vi "choosePathDS.vi"(8 "error in (no error)":errorcluster, 10 "ImagesTaken":i32, 11 "Pixelfly in":refnum<class "PixelflySA.lvclass">) -> (0 "error out":errorcluster, 2 "paths":path[](array[path]), 3 "Pixelfly out":refnum<class "PixelflySA.lvclass">)   [LabVIEW 2009, in "PixelflySA.lvclass"]
uses:
  PixelflySA.lvclass
  PixelflySA.lvclass/PixelflySA.ctl
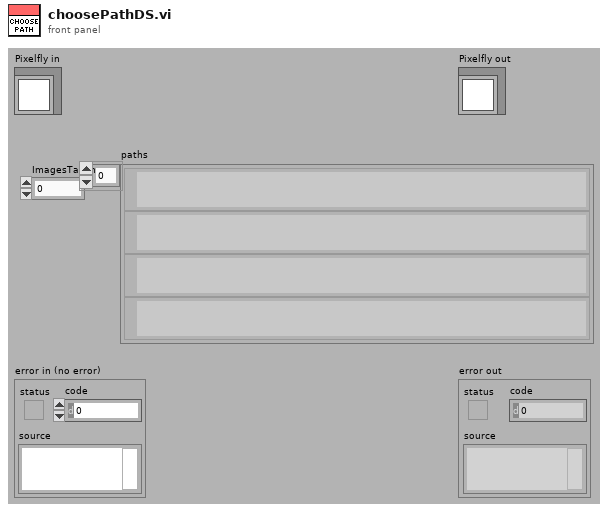
[diagram p1: front panel]
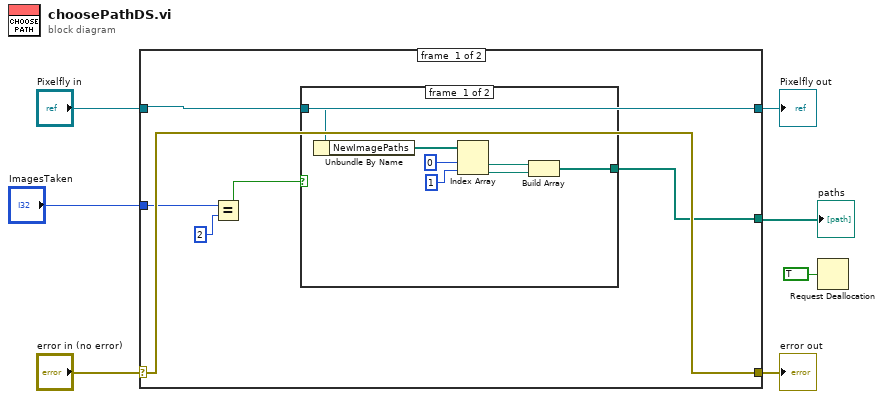
[diagram p0: block diagram]
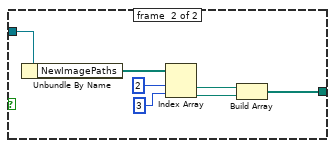
[diagram p2: hidden frame]
diagram:
  n1 = case shown="No Error" "error in (no error)" {
    selector: "error in (no error)" -> [w12 w29]
    tunnel: [w12 w29] -> w6
    tunnel: [w13 w28] -> w4
    tunnel: "Pixelfly in" -> [w13 w28]
    tunnel: [w9 _] -> w2
    tunnel: "ImagesTaken" -> [w10 _]
    frame #0 {
      n2 = Equal?(x=w10, y=2) -> (x = y?=w8:bool)
      n3 = case shown="True" w8 {
        tunnel: w13 -> [w20 w27]
        tunnel: [w14 w21] -> w9
        frame #0 {
          n4 = Unbundle By Name(w20) -> ("NewImagePaths"=w19:path[])
          n5 = Index Array(array=w19, index #1=0, index #2=1) -> (element #1=w16:path, element #2=w15:path)
          n6 = Build Array(w16, w15) -> (w14:path[])
        }
        frame #1 {
          n7 = Unbundle By Name(w27) -> ("NewImagePaths"=w26:path[])
          n8 = Index Array(array=w26, index #1=2, index #2=3) -> (element #1=w23:path, element #2=w22:path)
          n9 = Build Array(w23, w22) -> (w21:path[])
        }
      }
    }
    frame #1 {
    }
  }
  "error out" <- w6
  "Pixelfly out" <- w4
  "paths" <- w2
  n10 = Request Deallocation(TRUE ("flag")) -> ()
